vi "Read Graph Axis Labels (UTF-8 String).vi"(8 "error in":errorcluster, 11 "Control Ref":refnum<vi>) -> (0 "error out":errorcluster, 1 "Y Axis":refnum<class "UTF-8 String.lvclass">, 2 "X Axis":refnum<class "UTF-8 String.lvclass">)   [LabVIEW 2020, in "G-Unicode.lvlib"]
doc: "Reads text from a control or indicator, converting between encodings as necessary. <b>UTF-8 String</b> will be a scalar value, 1D array, or 2D array depending on <b>Control Ref</b> type.\n\nThe control text output will be converted to UTF-8 from either UTF-16LE or ANSI, depending on the control's Interpret As Unicode property or text Byte Order Mark (BOM).\n\nSupported control/indicator types and their outputs:\n- String (scalar)\n- String Array (1D)\n- String Array (2D)\n- Ring Text (1D)\n- Tab Pages (1D)\n- Boolean Text (1D, 4 elements)\n- Table (2D)\n- Listbox (1D)\n- Multicolumn Listbox (2D)"
uses:
  G-Unicode.lvlib
  f6f7f231-7ddf-476b-a943-0386d848a5c9.vi
  3fa1dd17-8c9f-4d8d-ac67-ec21dd2df23f.vi
  Types/UTF-8 String/UTF-8 String.lvclass
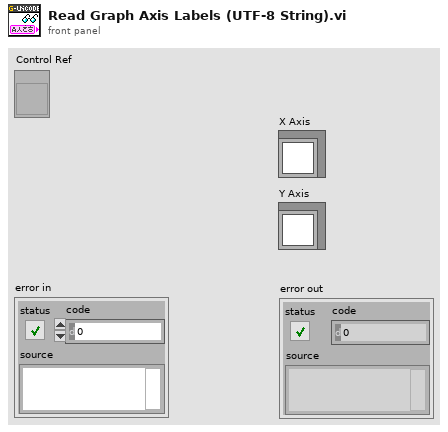
[diagram p1: front panel]
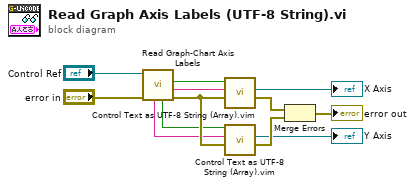
[diagram p0: block diagram]
diagram:
  n1 = call "Read Graph-Chart Axis Labels.vi"("error in"="error in", "Graph / Chart Reference in"="Control Ref") -> ("error out"=w7:errorcluster, "X Axis"=w9:string, "Interpret As Unicode (X)"=w10:bool, "Interpret As Unicode (Y)"=w5:bool, "Y Axis"=w6:string)  [unwired: 4 in, 1 out]
  n2 = call "Control Text as UTF-8 String (Array).vim"("Interpret As Unicode"=w10, "error in"=w7, "Control Text"=w9) -> ("error out"=w3:errorcluster, "UTF-8 String"=→"X Axis":refnum<class "UTF-8 String.lvclass">)  [unwired: 7 in]
  n3 = call "Control Text as UTF-8 String (Array).vim"("Interpret As Unicode"=w5, "error in"=w7, "Control Text"=w6) -> ("error out"=w4:errorcluster, "UTF-8 String"=→"Y Axis":refnum<class "UTF-8 String.lvclass">)  [unwired: 7 in]
  n4 = Merge Errors(w3, w4) -> (→"error out":errorcluster)
